vi "Read Representation.vi"(8 "error in (no error)":errorcluster, 11 "Scrollbar.lvclass in":refnum<class "Scrollbar.lvclass">) -> (0 "error out":errorcluster, 2 "Rep":T1, 3 "Scrollbar.lvclass out":refnum<class "Scrollbar.lvclass">)   [LabVIEW 2015, in "Scrollbar.lvclass"]
uses:
  Scrollbar.lvclass
  <vilib>/numeric/LVNumericRepresentation.ctl
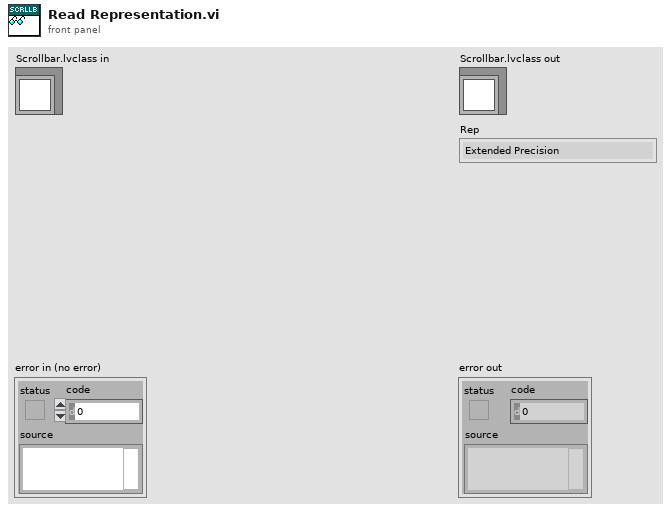
[diagram p1: front panel]
types:
  T1 = typedef "LVNumericRepresentation.ctl" = enum32{"Extended Precision", "Double Precision", "Single Precision", "Long", "Word", "Byte", "Unsigned Long", "Unsigned Word", "Unsigned Byte", "Complex Extended", "Complex Double", "Complex Single", "Quad", "Unsigned Quad", "Fixed-Point"}
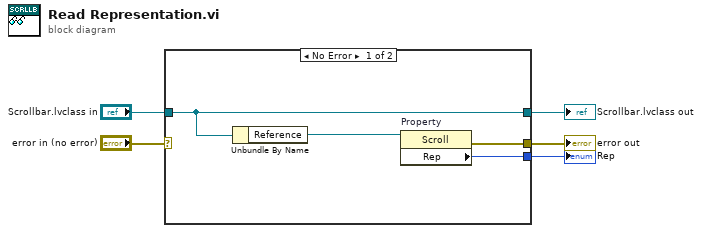
[diagram p0: block diagram]
diagram:
  n1 = case shown="No Error" "error in (no error)" {
    selector: "error in (no error)" -> [_ w11]
    tunnel: [w8 w11] -> w4
    tunnel: [w7 w10] -> w2
    tunnel: "Scrollbar.lvclass in" -> [w7 w10]
    tunnel: [w9 _] -> w1
    frame No Error {
      n2 = Unbundle By Name(w7) -> ("Reference"=w6:refnum<vi>)
      n3 = property on="Property" class="Scroll"(reference=w6) -> (error out=w8:errorcluster, "Rep"=w9:T1)  [unwired: 1 in, 1 out]
    }
    frame Error {
    }
  }
  "error out" <- w4
  "Scrollbar.lvclass out" <- w2
  "Rep" <- w1
